vi "SM Electrode Write To Buffer.vi"(4 "64-bitmask Input":u64 format="%064b", 5 "SM Electrode Grid Array":bool[][](array[boolean])=[[FALSE, FALSE, FALSE, FALSE, FALSE, FALSE], [FALSE, FALSE, FALSE, FALSE, FALSE, FALSE], [FALSE, FALSE, FALSE, FALSE, FALSE, FALSE], [FALSE, FALSE, FALSE, FALSE, FALSE, FALSE], [FALSE, FALSE, FALSE, FALSE, FALSE, FALSE], [FALSE, FALSE, FALSE, FALSE, FALSE, FALSE]]) -> (1 "64-bitmask Output":u64 format="%064b")   [LabVIEW 2017]
doc: "This VI will map the SM electrode grid array to ON-OFF bits in tehe 64 bit data buffer.\n\nAn array constant in this VI maps the SM electrode grid positions to the required HV channels."
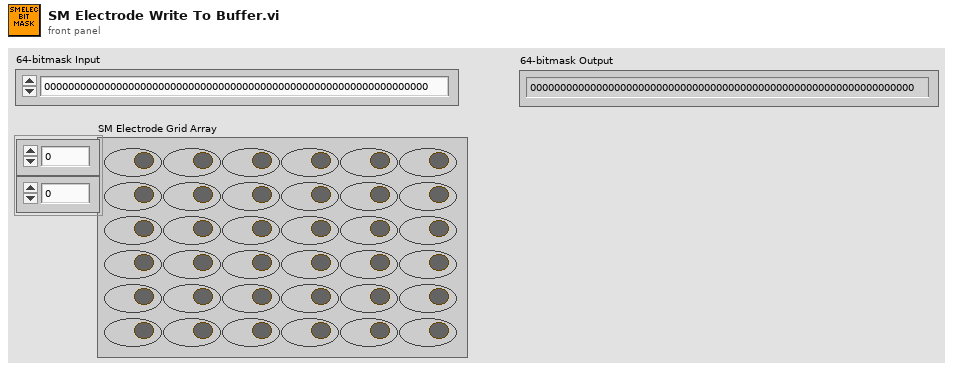
[diagram p1: front panel]
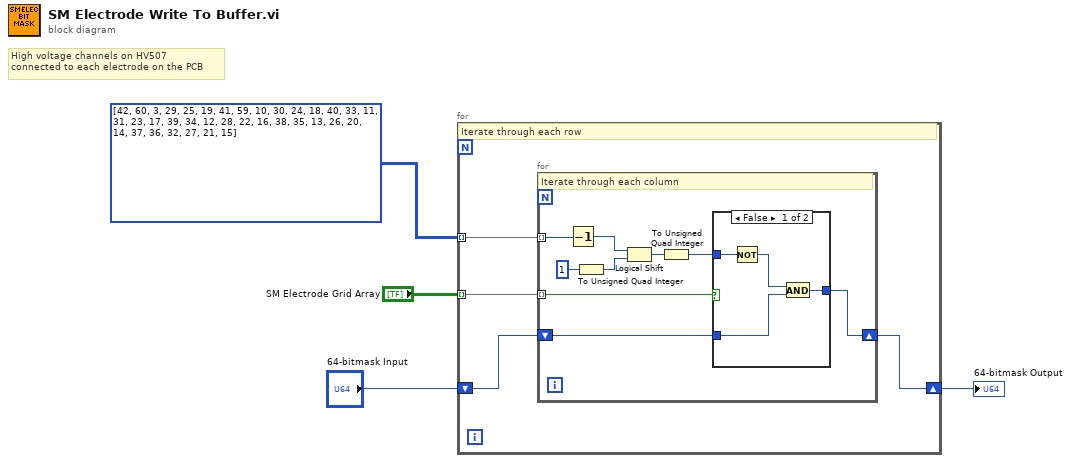
[diagram p0: block diagram]
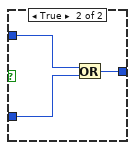
[diagram p2: hidden frame]
diagram:
  # "High voltage channels on HV507\nconnected to each electrode on the PCB"
  n1 = for {
    shift-right: [w7] -> w4
    shift-left: "64-bitmask Input" -> [w8]
    tunnel: "SM Electrode Grid Array" -> [w6] mode=indexing
    tunnel: u8[][] [[42, 60, 3, 29, 25, 19], [41, 59, 10, 30, 24, 18], [40, 33, 11, 31, 23, 17], [39, 34, 12, 28, 22, 16], [38, 35, 13, 26, 20, 14], [37, 36, 32, 27, 21, 15]] -> [w5] mode=indexing
    # "Iterate through each row"
    n2 = for {
      shift-right: [w15] -> w7
      shift-left: w8 -> [w10]
      tunnel: w6 -> [w11] mode=indexing
      tunnel: w5 -> [w13] mode=indexing
      # "Iterate through each column"
      n3 = Decrement(x=w13) -> (x-1=w12:u8)
      n4 = To Unsigned Quad Integer(1:u64 1 ("number")) -> (0:w14:u64)
      n5 = Logical Shift(y=w12, x=w14) -> (x << y=w17:u64)
      n6 = To Unsigned Quad Integer(1:w17) -> (0:w16:u64)
      n7 = case shown="False" w11 {
        tunnel: w16 -> [w21 w24]
        tunnel: [w18 w23] -> w15
        tunnel: w10 -> [w19 w22]
        frame False {
          n8 = Not(x=w21) -> (.not. x?=w20:u64)
          n9 = And(x=w20, y=w19) -> (x .and. y?=w18:u64)
        }
        frame True {
          n10 = Or(x=w24, y=w22) -> (x .or. y?=w23:u64)
        }
      }
    }
  }
  "64-bitmask Output" <- w4
